vi "send FPGA commands.vi"(6 "Message handler data":T1, 7 "RT Queues":T4, 11 "Data":variant) -> ()   [LabVIEW 2018]
uses:
  Type Defs/Message loop data.ctl
  Type Defs/FPGA reference.ctl
  Type Defs/RT Status.ctl
  Type Defs/Queues cluster.ctl
  ICL-LabVIEW_General/Message Scheduler/message scheduler.lvclass
  ICL-LabVIEW_General/Incident logger/Incidents/Warning/Warning.lvclass
  C:/GitHub/ICL-LabVIEW_General/Incident logger/Incidents/Incident.lvclass
  update digital outputs.vi
  update speed filter.vi
  update voltage outputs.vi
  update safe outputs.vi
  Queue VIs/En-queue RT FIFO element.vi
  Queue VIs/En-queue RT data element.vi
  Queue VIs/En-queue RT message element.vi
  restart FPGA.vi
panel:
  out "Message handler data 2":T1
  out "FPGA command":string
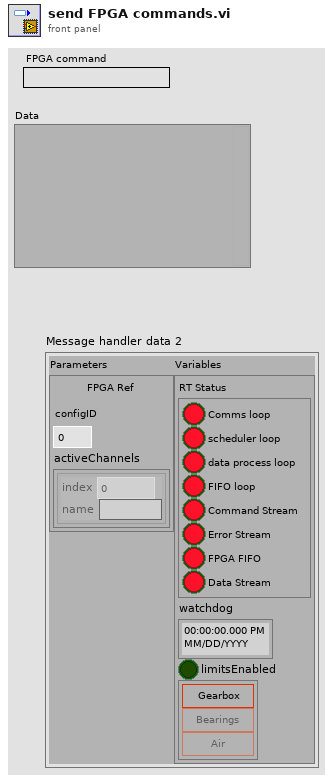
[diagram p1: front panel]
types:
  T1 = typedef "Message loop data.ctl" = cluster{"Parameters":cluster{"FPGA Ref":T2, "configID":u32, "activeChannels":cluster{"index":u16, "name":string}[]}, "Variables":cluster{"RT Status":T3, "watchdog":timestamp, "limitsEnabled":bool, "Interlocks":cluster{"gearboxOil":bool, "bearingOil":bool, "gearboxAir":bool}}}
  T2 = typedef "FPGA reference.ctl" = refnum<k20>
  T3 = typedef "RT Status.ctl" = cluster{"Comms loop":bool, "scheduler loop":bool, "data process loop":bool, "FIFO loop":bool, "Command Stream":bool, "Error Stream":bool, "FPGA FIFO":bool, "Data Stream":bool}
  T4 = typedef "Queues cluster.ctl" = cluster{"RT Message":refnum<queue>, "RT Comms":refnum<queue>, "RT Data":refnum<queue>, "RT FIFO":refnum<queue>, "message scheduler":refnum<class "message scheduler.lvclass">}
  T5 = cluster{"Target":string, "Loop":string, "Code":string}
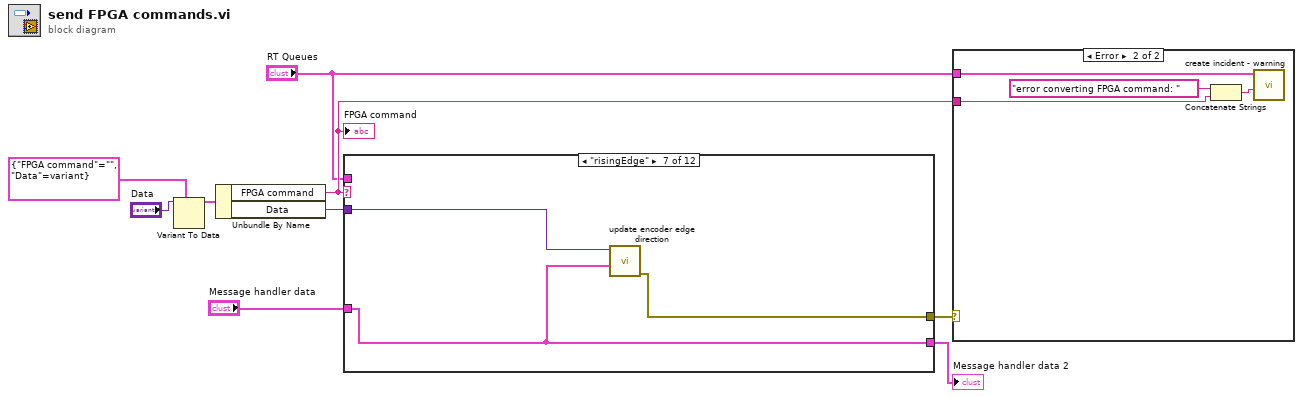
[diagram p0: block diagram]
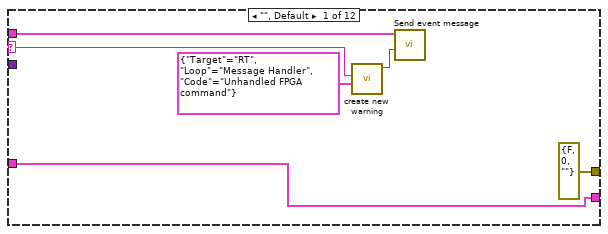
[diagram p3: hidden frame]
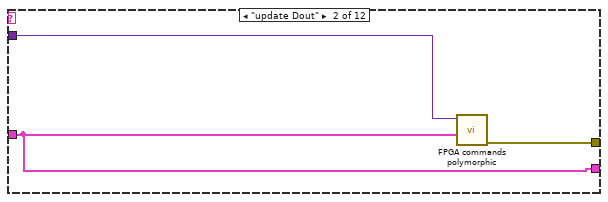
[diagram p4: hidden frame]
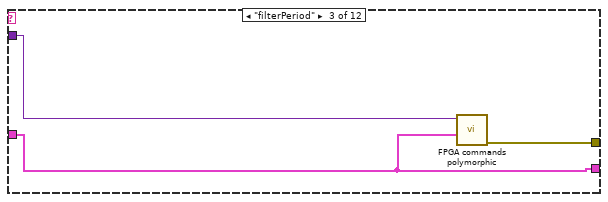
[diagram p5: hidden frame]
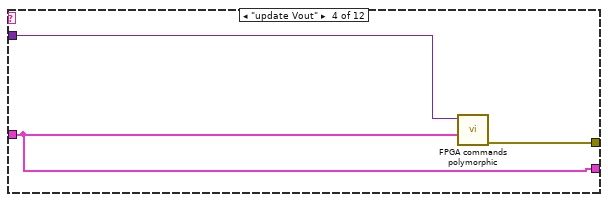
[diagram p6: hidden frame]
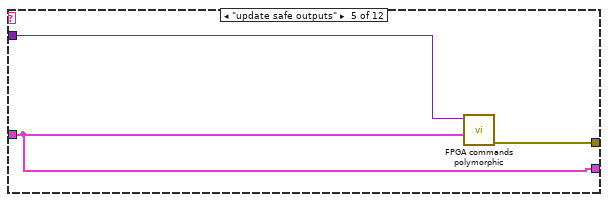
[diagram p7: hidden frame]
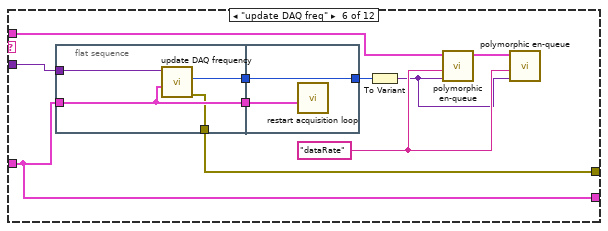
[diagram p8: hidden frame]
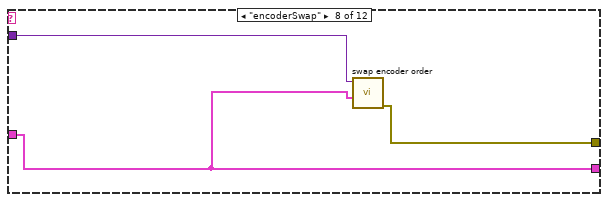
[diagram p9: hidden frame]
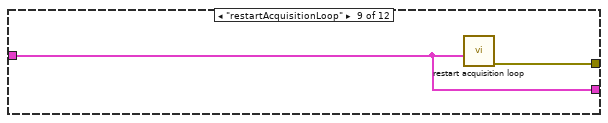
[diagram p10: hidden frame]
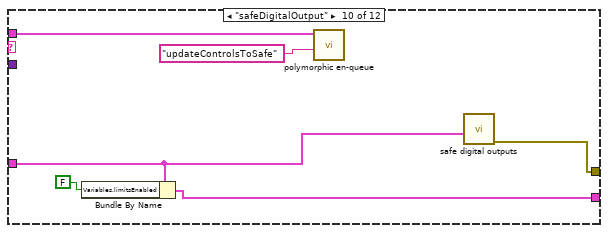
[diagram p11: hidden frame]
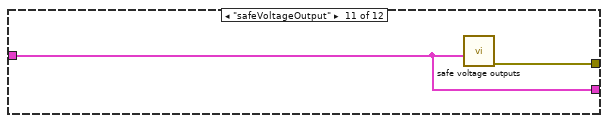
[diagram p12: hidden frame]
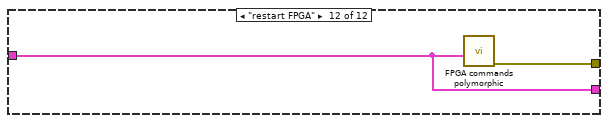
[diagram p13: hidden frame]
diagram:
  n1 = Variant To Data(type=cluster{"FPGA command":string, "Data":variant} {"FPGA command"="", "Data"=variant}, Variant="Data") -> (data=w9:cluster{"FPGA command":string, "Data":variant})  [unwired: 1 in, 1 out]
  n2 = Unbundle By Name(w9) -> ("FPGA command"=w3:string, "Data"=w6:variant)
  "FPGA command" <- w3
  n3 = case shown="\"risingEdge\"" w3 {
    selector: w3 -> [w14 _ _ _ _ _ _ _ _ _ _ _]
    tunnel: w6 -> [_ w18 w21 w24 w27 w37 w46 w49 _ _ _ _]
    tunnel: "Message handler data" -> [w10 w16 w20 w22 w25 w36 w45 w48 w50 w56 w58 w60]
    tunnel: [errorcluster {"status"=FALSE, "code"=0, "source"=""} ("variant error") w17 w19 w23 w26 w34 w44 w47 w51 w57 w59 w61] -> w4
    tunnel: "RT Queues" -> [w13 _ _ _ _ w32 _ _ _ w53 _ _]
    tunnel: [w10 w16 w20 w22 w25 w36 w45 w48 w50 w55 w58 w60] -> w1
    frame "", Default {
      n4 = call "create new warning.vi"("Location"=T5 {"Target"="RT", "Loop"="Message Handler", "Code"="Unhandled FPGA command"}, "Description"=w14) -> ("Warning out"=w15:refnum<class "Warning.lvclass">)  [unwired: 8 in, 1 out]
      n5 = call "Send event message.vi"("Incident"=w15, "RT Queues"=w13) -> ()  [unwired: 9 in, 1 out]
    }
    frame "update Dout" {
      n6 = call-poly "FPGA commands polymorphic.vi"("Message handler data"=w16, "Data"=w18) -> ("error"=w17:errorcluster)  [unwired: 9 in]
    }
    frame "filterPeriod" {
      n7 = call-poly "FPGA commands polymorphic.vi"("Message handler data"=w20, "Data"=w21) -> ("variant error"=w19:errorcluster)  [unwired: 9 in]
    }
    frame "update Vout" {
      n8 = call-poly "FPGA commands polymorphic.vi"("Message handler data"=w22, "Data"=w24) -> ("error out"=w23:errorcluster)  [unwired: 9 in]
    }
    frame "update safe outputs" {
      n9 = call-poly "FPGA commands polymorphic.vi"("Message handler data"=w25, "Data"=w27) -> ("error"=w26:errorcluster)  [unwired: 9 in]
    }
    frame "update DAQ freq" {
      w29 = "dataRate" ("Message")
      n10 = flat-sequence {
        tunnel: w37 -> [w41]
        tunnel: w36 -> [w40]
        tunnel: [w40] -> w35
        tunnel: [w39] -> w34
        tunnel: [w38] -> w33
        tunnel: w35 -> [w43]
        tunnel: w33 -> [w42]
        tunnel: [w42] -> w31
        frame #0 {
          n11 = call "update DAQ frequency.vi"("Message handler data"=w40, "Data"=w41) -> ("variant error"=w39:errorcluster, "dataRate"=w38:u16)  [unwired: 8 in]
        }
        frame #1 {
          n12 = call "restart acquisition loop.vi"("Message handler data"=w43) -> ()  [unwired: 10 in, 1 out]
        }
      }
      n13 = To Variant(anything=w31) -> (Variant=w28:variant)
      n14 = call-poly "polymorphic en-queue.vi"("Data"=w28, "Message"=w29, "RT Queues"=w32) -> ("RT Queues out"=w30:T4)  [unwired: 6 in, 2 out]
      n15 = call-poly "polymorphic en-queue.vi"("Data"=w28, "Message"=w29, "RT Queues"=w30) -> ()  [unwired: 6 in, 3 out]
    }
    frame "risingEdge" {
      n16 = call "update encoder edge direction.vi"("Message handler data"=w45, "Data"=w46) -> ("variant error"=w44:errorcluster)  [unwired: 9 in]
    }
    frame "encoderSwap" {
      n17 = call "swap encoder order.vi"("Message handler data"=w48, "Data"=w49) -> ("variant error"=w47:errorcluster)  [unwired: 9 in]
    }
    frame "restartAcquisitionLoop" {
      n18 = call "restart acquisition loop.vi"("Message handler data"=w50) -> ("error out"=w51:errorcluster)  [unwired: 10 in]
    }
    frame "safeDigitalOutput" {
      n19 = Bundle By Name(cluster=w56, "Variables.limitsEnabled"=FALSE) -> (w55:T1)
      n20 = call-poly "polymorphic en-queue.vi"("Message"="updateControlsToSafe", "RT Queues"=w53) -> ()  [unwired: 9 in, 1 out]
      n21 = call "safe digital outputs.vi"("Message handler data"=w56) -> ("error out"=w57:errorcluster)  [unwired: 10 in]
    }
    frame "safeVoltageOutput" {
      n22 = call "safe voltage outputs.vi"("Message handler data"=w58) -> ("error out"=w59:errorcluster)  [unwired: 10 in]
    }
    frame "restart FPGA" {
      n23 = call-poly "FPGA commands polymorphic.vi"("Message handler data"=w60) -> ("error out"=w61:errorcluster)  [unwired: 10 in]
    }
  }
  "Message handler data 2" <- w1
  n24 = case shown="Error" w4 {
    tunnel: "RT Queues" -> [_ w65]
    tunnel: w3 -> [_ w62]
    frame No Error {
    }
    frame Error {
      n25 = Concatenate Strings("error converting FPGA command: " ("Description"), w62) -> (w63:string)
      n26 = call "create incident - warning.vi"("warning description"=w63, "RT Queues"=w65) -> ()  [unwired: 9 in, 1 out]
    }
  }
